vi "UsrProfiles-Import profile.vi"   [LabVIEW 2013]
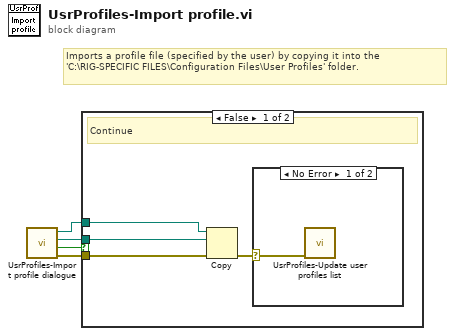
[diagram p0: block diagram]
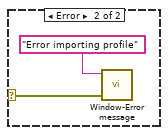
[diagram p2: hidden frame]
diagram:
  # "Imports a profile file (specified by the user) by copying it into the\n'C:\\RIG-SPECIFIC FILES\\Configuration Files\\User Profiles' folder."
  n1 = call "UsrProfiles-Import profile dialogue.vi"() -> ("error out"=w4:errorcluster, "cancelled"=w3:bool, "target filepath"=w2:path, "Source filepath"=w1:path)  [unwired: 8 in]
  n2 = case shown="False" w3 {
    tunnel: w1 -> [w6 _]
    tunnel: w2 -> [w8 _]
    tunnel: w4 -> [w7 _]
    frame False {
      # "Continue"
      n3 = Copy(8:w7, 10:w8, 11:w6) -> (0:w5:errorcluster)  [unwired: 2 in, 2 out]
      n4 = case shown="No Error" w5 {
        selector: w5 -> [w9 w11]
        frame No Error {
          n5 = call "UsrProfiles-Update user profiles list.vi"("error in"=w9) -> ()  [unwired: 10 in, 1 out]
        }
        frame Error {
          n6 = call "Window-Error message.vi"("error in (no error)"=w11, "Message"="Error importing profile") -> ()  [unwired: 9 in, 1 out]
        }
      }
    }
    frame True {
      # "Cancelled"
    }
  }
